vi "Initialise.vi"(8 "error in (no error)":errorcluster, 10 "Message in":refnum<class "InitialiseMessage.lvclass">, 11 "waveform_FPGA in":refnum<class "waveform_FPGA.lvclass">) -> (0 "error out":errorcluster, 3 "waveform_FPGA out":refnum<class "waveform_FPGA.lvclass">)   [LabVIEW 2012, in "waveform_FPGA.lvclass"]
doc: "This method is called when an initialise message is received. It mainly initialises the RabbitMQ connectivity. \n\nOverride this method when your component needs special initialisation (e.g. of software or hardware resources). In that case, don't forget to call the parent for proper implementation. If your component owns subcomponents, they count as resources, so you have to initialise them by calling their own initialise functions"
uses:
  waveform_FPGA.lvclass
  <vilib>/Distrio/Murmex/Murmex/Murmex.lvclass
  <vilib>/Distrio/Murmex/InitialiseMessage/InitialiseMessage.lvclass
panel:
  # "This method is called when the INTIALISE\ntrigger is sent. \n\nOverride this method when your component needs to\nrespond to this trigger. \n\nCall parent for proper implementation"
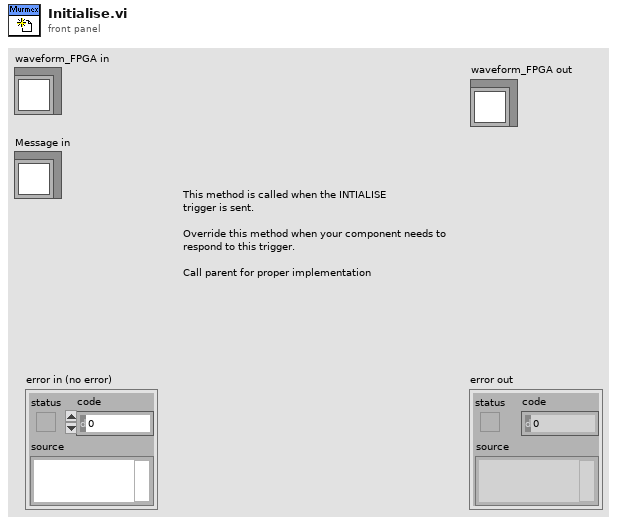
[diagram p1: front panel]
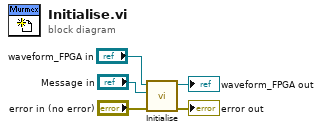
[diagram p0: block diagram]
diagram:
  n1 = call-parent "Initialise.vi"("error in (no error)"="error in (no error)", "Message in"="Message in", "Murmex in"="waveform_FPGA in") -> ("error out"=→"error out":errorcluster, "Murmex out"=→"waveform_FPGA out":refnum<class "waveform_FPGA.lvclass">)  [unwired: 7 in]
